vi "STOP_ALL.vi"(10 "argv":string[](array[string]), 11 "args":u8) -> ()   [LabVIEW 2014]
uses:
  TORC Code/GlobalVariable.vi
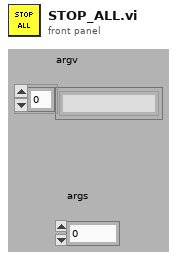
[diagram p1: front panel]
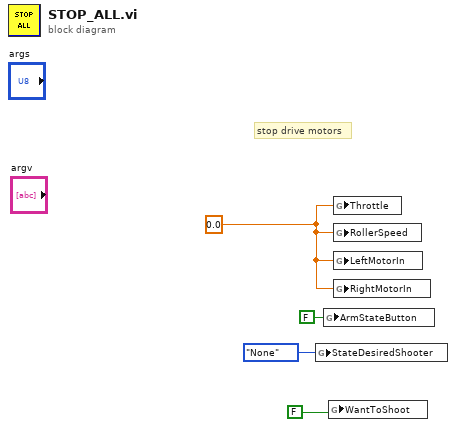
[diagram p0: block diagram]
diagram:
  w4 = 0.0 ("Left Motor")
  # "stop drive motors"
  n1 = global write "GlobalVariable.vi" "StateDesiredShooter"(enum16{"None", "Down", "Up"}."None" ("StateDesiredShooter")) -> ()
  n2 = global write "GlobalVariable.vi" "ArmStateButton"(FALSE ("ArmStateButton")) -> ()
  n3 = global write "GlobalVariable.vi" "WantToShoot"(FALSE ("WantToShoot")) -> ()
  n4 = global write "GlobalVariable.vi" "Throttle"(w4) -> ()
  n5 = global write "GlobalVariable.vi" "RollerSpeed"(w4) -> ()
  n6 = global write "GlobalVariable.vi" "LeftMotorIn"(w4) -> ()
  n7 = global write "GlobalVariable.vi" "RightMotorIn"(w4) -> ()
